vi "Write Status.vi"(8 "error in (no error)":errorcluster, 10 "Status":T1, 11 "Image Processing Handler in":refnum<class "Image Processing Handler.lvclass">) -> (0 "error out":errorcluster, 3 "Image Processing Handler out":refnum<class "Image Processing Handler.lvclass">)   [LabVIEW 2018, in "Image Processing Handler.lvclass"]
uses:
  Image Processing Handler.lvclass
  Video Frame/Video Frame.lvclass
  Image Processing Handler.lvclass/Image Processing Handler.ctl
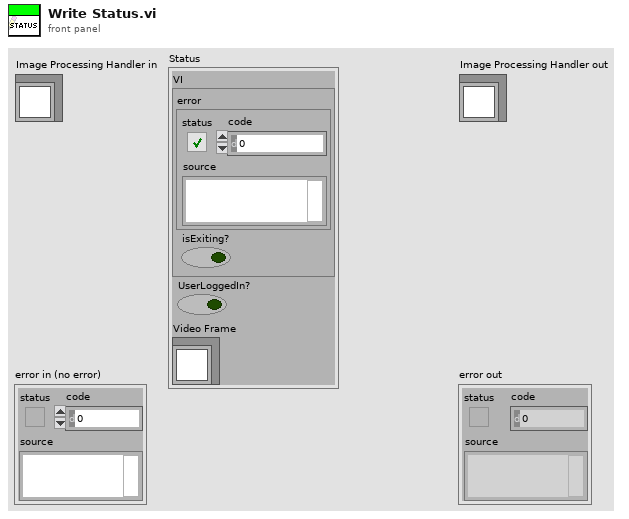
[diagram p1: front panel]
types:
  T1 = cluster{"VI":cluster{"error":errorcluster, "isExiting?":bool}, "UserLoggedIn?":bool, "Video Frame":refnum<class "Video Frame.lvclass">}
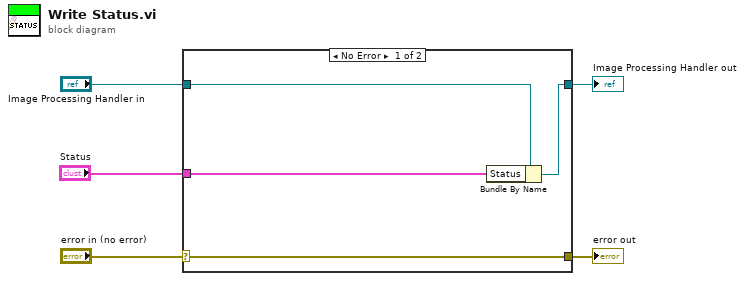
[diagram p0: block diagram]
diagram:
  n1 = case shown="No Error" "error in (no error)" {
    selector: "error in (no error)" -> [w9 w10]
    tunnel: [w9 w10] -> w4
    tunnel: [w7 w11] -> w2
    tunnel: "Image Processing Handler in" -> [w8 w11]
    tunnel: "Status" -> [w6 _]
    frame No Error {
      n2 = Bundle By Name(cluster=w8, "Status"=w6) -> (w7:refnum<class "Image Processing Handler.lvclass">)
    }
    frame Error {
    }
  }
  "error out" <- w4
  "Image Processing Handler out" <- w2
